vi "Wrap Position.vi"(11 "Motion in":refnum<class "Motion.lvclass">) -> (3 "Motion out":refnum<class "Motion.lvclass">)   [LabVIEW 2021, in "Motion.lvclass"]
uses:
  Motion.lvclass
  Motion.lvclass/Motion.ctl
  Vector 2D/Vector 2D.lvclass
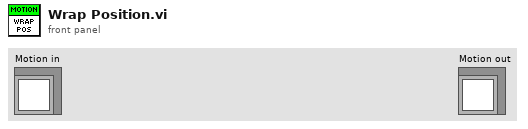
[diagram p1: front panel]
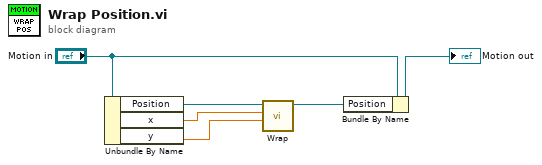
[diagram p0: block diagram]
diagram:
  n1 = Unbundle By Name("Motion in") -> ("Position"=w4:refnum<class "Vector 2D.lvclass">, "x"=w2:sgl, "y"=w1:sgl)
  n2 = call "Wrap.vi"("Max y"=w1, "Max x"=w2, "Vector 2D in"=w4) -> ("Vector 2D out"=w3:refnum<class "Vector 2D.lvclass">)  [unwired: 8 in]
  n3 = Bundle By Name(cluster="Motion in", "Position"=w3) -> (→"Motion out":refnum<class "Motion.lvclass">)
